vi "Storage Command Handler Test.vi"(6 "Operator POVs":i16[](array[numeric]), 7 "Driver POVs":i16[](array[numeric]), 8 "Operator Axes":dbl[](array[numeric]), 9 "Operator Buttons":bool[](array[boolean]), 10 "Driver Buttons":bool[](array[boolean]), 11 "Driver Axes":dbl[](array[numeric])) -> ()   [LabVIEW 2019]
uses:
  cf9eb55e-d57c-46e7-9f03-3df8d9565ed4.vi
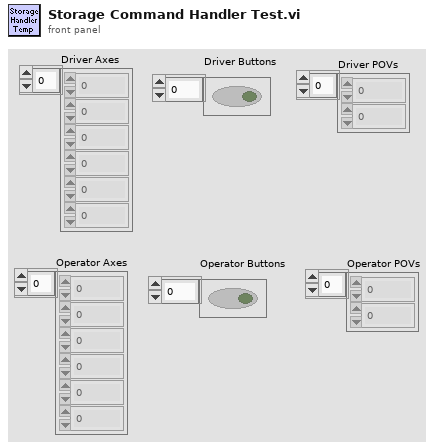
[diagram p1: front panel]
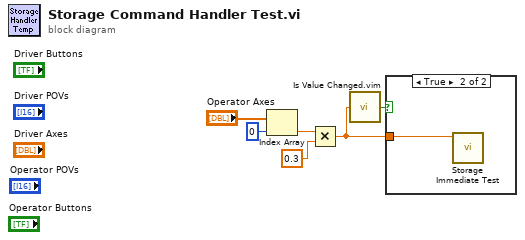
[diagram p0: block diagram]
diagram:
  n1 = Index Array(array="Operator Axes", index=0) -> (element=w4:dbl)
  n2 = Multiply(x=w4, y=0.3) -> (x*y=w2:dbl)
  n3 = call "Is Value Changed.vim"("value"=w2) -> ("changed or first call?"=w1:bool)
  n4 = case shown="True" w1 {
    tunnel: w2 -> [_ w7]
    frame False {
    }
    frame True {
      n5 = call "Storage Immediate Test.vi"("Setpoint"=w7) -> ()  [unwired: 10 in, 1 out]
    }
  }
